vi "Shorten Call Chain to Length.vi"(9 "desired length":i32, 10 "delimiter":string, 11 "call chain in":string[](array[string])) -> (3 "call chain out":string[](array[string]))   [LabVIEW 2024, in "Logging.lvlib" / "Format String.lvclass"]
uses:
  Format String.lvclass
  Utilities/Utilities.lvlib
panel:
  # "Connector Pane"
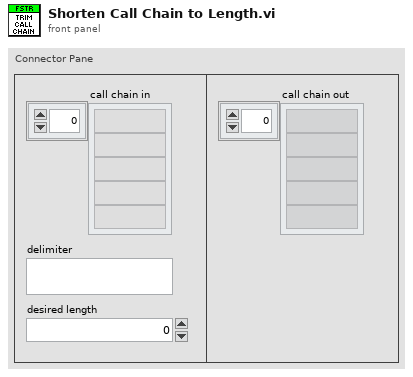
[diagram p1: front panel]
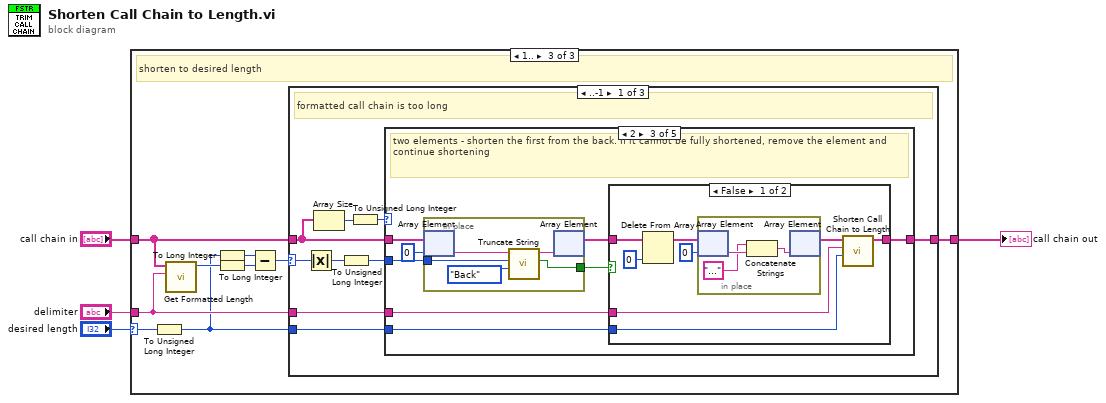
[diagram p0: block diagram]
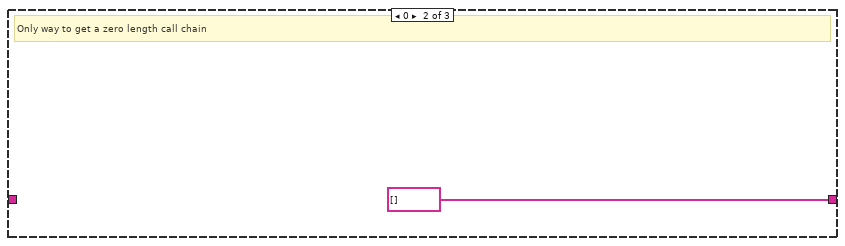
[diagram p3: hidden frame]
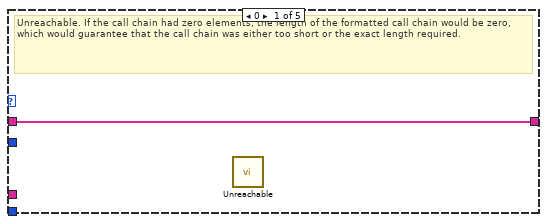
[diagram p4: hidden frame]
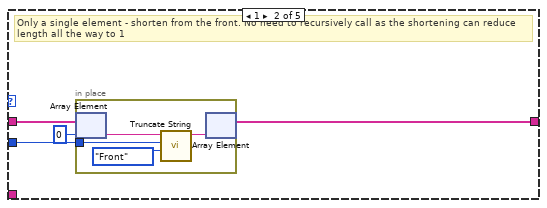
[diagram p5: hidden frame]
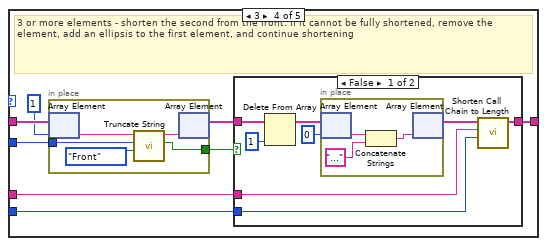
[diagram p7: hidden frame]
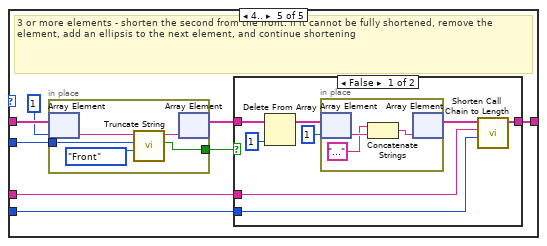
[diagram p9: hidden frame]
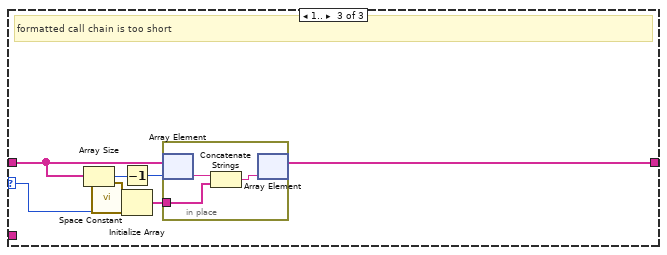
[diagram p12: hidden frame]
diagram:
  n1 = case shown="1.." "desired length" {
    selector: "desired length" -> [_ _ w10]
    tunnel: "delimiter" -> [_ _ w15]
    tunnel: "call chain in" -> [w5 _ w14]
    tunnel: [w5 string[] [] ("call chain in") w13] -> w2
    frame ..-1 {
      # "negative length - skip and leave as-is"
    }
    frame 0 {
      # "Only way to get a zero length call chain"
    }
    frame 1.. {
      # "shorten to desired length"
      n2 = To Unsigned Long Integer(number=w10) -> (unsigned 32bit integer=w9:u32)
      n3 = call "Get Formatted Length.vi"("delimiter"=w15, "call chain"=w14) -> ("formatted length"=w11:u32)  [unwired: 9 in]
      n4 = To Long Integer(number=w9) -> (32bit integer=w8:i32)
      n5 = To Long Integer(number=w11) -> (32bit integer=w7:i32)
      n6 = Subtract(x=w8, y=w7) -> (x-y=w12:i32)
      n7 = case shown="..-1" w12 {
        selector: w12 -> [w22 _ w110]
        tunnel: w14 -> [w23 w109 w115]
        tunnel: [w20 w109 w111] -> w13
        tunnel: w15 -> [w18 _ _]
        tunnel: w9 -> [w17 _ _]
        frame ..-1 {
          # "formatted call chain is too long"
          n8 = Absolute Value(x=w22) -> (abs(x)=w21:i32)
          n9 = Array Size(array=w23) -> (size(s)=w24:i32)
          n10 = To Unsigned Long Integer(number=w21) -> (unsigned 32bit integer=w19:u32)
          n11 = To Unsigned Long Integer(number=w24) -> (unsigned 32bit integer=w16:u32)
          n12 = case shown="2" w16 {
            tunnel: w23 -> [w25 w29 w41 w64 w89]
            tunnel: w19 -> [_ w28 w40 w61 w86]
            tunnel: [w25 w27 w37 w63 w88] -> w20
            tunnel: w18 -> [_ _ w35 w60 w85]
            tunnel: w17 -> [_ _ w36 w59 w84]
            frame 0 {
              # "Unreachable. If the call chain had zero elements, the length of the formatted call chain would be zero, which would guarantee that the call chain was either too short or the exact length required."
              n13 = call "Unreachable.vi"() -> ()  [unwired: 12 in]
            }
            frame 1 {
              # "Only a single element - shorten from the front. No need to recursively call as the shortening can reduce length all the way to 1"
              n14 = in-place {
                in-place-border: w28 -> [w32]
                n15 = in-place-array #1(w29, 0) -> (w33:string)
                n16 = call "Truncate String.vi"("direction"=enum16{"Front", "Back"}."Front", "# of characters to remove"=w32, "string"=w33) -> ("truncated string"=w31:string)  [unwired: 7 in, 1 out]
                n17 = in-place-array #1(w31) -> (w27:string[])  [unwired: 1 out]
              }
            }
            frame 2 {
              # "two elements - shorten the first from the back. If it cannot be fully shortened, remove the element and continue shortening"
              n18 = in-place {
                in-place-border: w40 -> [w57]
                in-place-border: [w54] -> w38
                n19 = in-place-array #2(w41, 0) -> (w58:string)
                n20 = call "Truncate String.vi"("direction"=enum16{"Front", "Back"}."Back", "# of characters to remove"=w57, "string"=w58) -> ("removed all?"=w54:bool, "truncated string"=w56:string)  [unwired: 7 in]
                n21 = in-place-array #2(w56) -> (w39:string[])  [unwired: 1 out]
              }
              n22 = case shown="False" w38 {
                tunnel: w39 -> [w49 w53]
                tunnel: [w47 w53] -> w37
                tunnel: w36 -> [w46 _]
                tunnel: w35 -> [w45 _]
                frame False {
                  n23 = Delete From Array(array=w49, index=0) -> (array with subset deleted=w43:string[])  [unwired: 1 in, 1 out]
                  n24 = in-place {
                    n25 = in-place-array #3(w43, 0) -> (w52:string)
                    n26 = Concatenate Strings("…", w52) -> (w50:string)
                    n27 = in-place-array #3(w50) -> (w42:string[])  [unwired: 1 out]
                  }
                  n28 = call "Shorten Call Chain to Length.vi"("desired length"=w46, "delimiter"=w45, "call chain in"=w42) -> ("call chain out"=w47:string[])  [unwired: 8 in]
                }
                frame True {
                }
              }
            }
            frame 3 {
              # "3 or more elements - shorten the second from the front. If it cannot be fully shortened, remove the element, add an ellipsis to the first element, and continue shortening"
              n29 = in-place {
                in-place-border: w61 -> [w82]
                in-place-border: [w79] -> w65
                n30 = in-place-array #4(w64, 1) -> (w83:string)
                n31 = call "Truncate String.vi"("direction"=enum16{"Front", "Back"}."Front", "# of characters to remove"=w82, "string"=w83) -> ("removed all?"=w79:bool, "truncated string"=w81:string)  [unwired: 7 in]
                n32 = in-place-array #4(w81) -> (w66:string[])  [unwired: 1 out]
              }
              n33 = case shown="False" w65 {
                tunnel: w66 -> [w74 w78]
                tunnel: [w72 w78] -> w63
                tunnel: w59 -> [w71 _]
                tunnel: w60 -> [w70 _]
                frame False {
                  n34 = Delete From Array(array=w74, index=1) -> (array with subset deleted=w69:string[])  [unwired: 1 in, 1 out]
                  n35 = in-place {
                    n36 = in-place-array #5(w69, 0) -> (w77:string)
                    n37 = Concatenate Strings(w77, "…") -> (w75:string)
                    n38 = in-place-array #5(w75) -> (w67:string[])  [unwired: 1 out]
                  }
                  n39 = call "Shorten Call Chain to Length.vi"("desired length"=w71, "delimiter"=w70, "call chain in"=w67) -> ("call chain out"=w72:string[])  [unwired: 8 in]
                }
                frame True {
                }
              }
            }
            frame 4.. {
              # "3 or more elements - shorten the second from the front. If it cannot be fully shortened, remove the element, add an ellipsis to the next element, and continue shortening"
              n40 = in-place {
                in-place-border: w86 -> [w107]
                in-place-border: [w104] -> w90
                n41 = in-place-array #6(w89, 1) -> (w108:string)
                n42 = call "Truncate String.vi"("direction"=enum16{"Front", "Back"}."Front", "# of characters to remove"=w107, "string"=w108) -> ("removed all?"=w104:bool, "truncated string"=w106:string)  [unwired: 7 in]
                n43 = in-place-array #6(w106) -> (w91:string[])  [unwired: 1 out]
              }
              n44 = case shown="False" w90 {
                tunnel: w91 -> [w99 w103]
                tunnel: [w97 w103] -> w88
                tunnel: w84 -> [w96 _]
                tunnel: w85 -> [w95 _]
                frame False {
                  n45 = Delete From Array(array=w99, index=1) -> (array with subset deleted=w94:string[])  [unwired: 1 in, 1 out]
                  n46 = in-place {
                    n47 = in-place-array #7(w94, 1) -> (w102:string)
                    n48 = Concatenate Strings("…", w102) -> (w100:string)
                    n49 = in-place-array #7(w100) -> (w92:string[])  [unwired: 1 out]
                  }
                  n50 = call "Shorten Call Chain to Length.vi"("desired length"=w96, "delimiter"=w95, "call chain in"=w92) -> ("call chain out"=w97:string[])  [unwired: 8 in]
                }
                frame True {
                }
              }
            }
          }
        }
        frame 0 {
          # "formatted call chain is exactly the correct length."
        }
        frame 1.. {
          # "formatted call chain is too short"
          n51 = Array Size(array=w115) -> (size(s)=w116:i32)
          n52 = call <vilib>:"Space Constant.vi"() -> ("String"=w113:string)
          n53 = Decrement(x=w116) -> (x-1=w114:i32)
          n54 = Initialize Array(w113, w110) -> (w112:string[])
          n55 = in-place {
            in-place-border: w112 -> [w118]
            n56 = in-place-array #8(w115, w114) -> (w119:string)
            n57 = Concatenate Strings(w119, w118) -> (w117:string)
            n58 = in-place-array #8(w117) -> (w111:string[])  [unwired: 1 out]
          }
        }
      }
    }
  }
  "call chain out" <- w2
